vi "Loopback FPGA.vi"() -> ()   [LabVIEW 2013]
uses:
  <vilib>/Platform/TimedLoop/XDataNode/timing_clust.ctl
  <vilib>/Platform/TimedLoop/XDataNode/nitl_modes.ctl
  <vilib>/Platform/TimedLoop/XDataNode/wakeup.ctl
  <vilib>/NI/I2S-TDM IP/Controls/transmitter configuration.ctl
  <vilib>/NI/I2S-TDM IP/Controls/sync modes.ctl
  <vilib>/NI/I2S-TDM IP/Controls/receiver configuration.ctl
  <vilib>/rvi/DataTransferAndStorage/Container/Common/niFpgaContainerGetUniqueNameForEmu.vi
  <vilib>/rvi/DataTransferAndStorage/Container/Common/niFpgaContainerSetEmuInfo.vi
  <vilib>/rvi/eio/common/nirviEmuReportErrorAndStop.vi
  <vilib>/rvi/Emulation/niFpgaSctlEmulationGetInTimedLoop.vi
  <vilib>/rvi/Emulation/niFpgaEmulationReportErrorSimple.vi
  <vilib>/rvi/Emulation/niFpgaGetClockAttributes.vi
  <vilib>/rvi/Emulation/niFpgaCriticalErrorInLSC.vi
  <vilib>/rvi/DataTransferAndStorage/Container/Common/niFpgaContainerExecOnDevCompGetState.vi
  <vilib>/rvi/FIFO/Fifo_Resource/nirvififoEmulationReadFpgaImpl.vi
  <vilib>/rvi/interface/RandomDataEmulation/nirviRandomDataFPGAFIFO.vi
  <vilib>/rvi/interface/RandomDataEmulation/niFpgaRandomDataHandleErrors.vi
  <vilib>/rvi/FIFO/Fifo_Resource/nirvififoEmulationGetNumberOfElementsToReadFpgaImpl.vi
  <vilib>/rvi/FIFO/Fifo_Resource/nirvififoEmulationWriteFpgaImpl.vi
  <vilib>/rvi/FIFO/Fifo_Resource/nirvififoEmulationGetNumberOfElementsToWriteFpgaImpl.vi
  <vilib>/Platform/TimedLoop/XDataNode/XDataNode.xnode
  <vilib>/rvi/LocalResourceManager/LocalResourceManager.xnode
  <vilib>/rvi/DataTransferAndStorage/Container/XNode/niFpgaContainer.xnode
  <vilib>/rvi/FIFO/Fifo_Resource/niFpgaFifoEmulationRefIn.vi
  <vilib>/NI/I2S-TDM IP/I2S-TDM.lvlib
  <vilib>/Platform/TimedLoop/XDataNode/XDNodeRunTimeDep.lvlib
panel:
  in  "samples in":u32[](array[numeric])=[0, 0, 0, 0, 0, 0, 0, 0]
  out "receive buffer":u32
  out "signals out":cluster{"clock":bool, "sync":bool, "sdata":bool}
  out "samples out":u32[](array[numeric])
  out "transmit buffer":u32
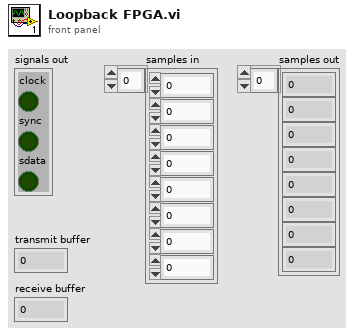
[diagram p1: front panel]
types:
  T1 = typedef "XDNodeRunTimeDep.lvlib/timing_clust.ctl" = cluster{"Expected End [f-1]":u64, "Actual End [f-1]":u64, "Finished Late? [f-1]":bool, "Expected End [i-1]":u64, "Actual End [i-1]":u64, "Finished Late? [i-1]":bool, "Expected Start [i]":u64, "Actual Start [i]":u64, "Expected Start [f]":u64, "Actual Start [f]":u64, "Source Name":string, "Structure Name":string, "Period":i64, "Deadline":i64, "Offset":i64, "Start":i64, "Priority":i32, "Timeout":i32, "Mode":T2, "Wakeup Reason":T3, "Error":errorcluster, "Source Type":string, "Secondary Source Type":string, "Global End Time":u64, "Global Start Time":u64, "Frame Duration":u64, "Iteration Duration":u64, "Assigned CPU":i32, "I/O Scan Engine Mode":u32}
  T2 = typedef "XDNodeRunTimeDep.lvlib/nitl_modes.ctl" = enum32{"No Change", "Process missed periods, maintain original phase", "Discard missed periods, maintain original phase", "Process missed periods, ignore original phase", "Discard missed periods, ignore original phase"}
  T3 = typedef "XDNodeRunTimeDep.lvlib/wakeup.ctl" = enum32{"Normal", "Aborted", "Asynchronous wakeup", "Timing source error", "Timed loop error", "Timeout"}
  T4 = typedef "I2S-TDM.lvlib/transmitter configuration.ctl" = cluster{"number of channels":u8, "bits per channel":u8, "data set edge":enum16{"rising", "falling"}, "sync mode":T5, "invert sync":bool}
  T5 = typedef "I2S-TDM.lvlib/sync modes.ctl" = enum16{"TDM - Sample Clock", "TDM - Pre-Start Pulse"}
  T6 = typedef "I2S-TDM.lvlib/receiver configuration.ctl" = cluster{"number of channels":u8, "bits per channel":u8, "data sample edge":enum16{"rising", "falling"}, "frame start delay":u8, "inverted sync":bool}
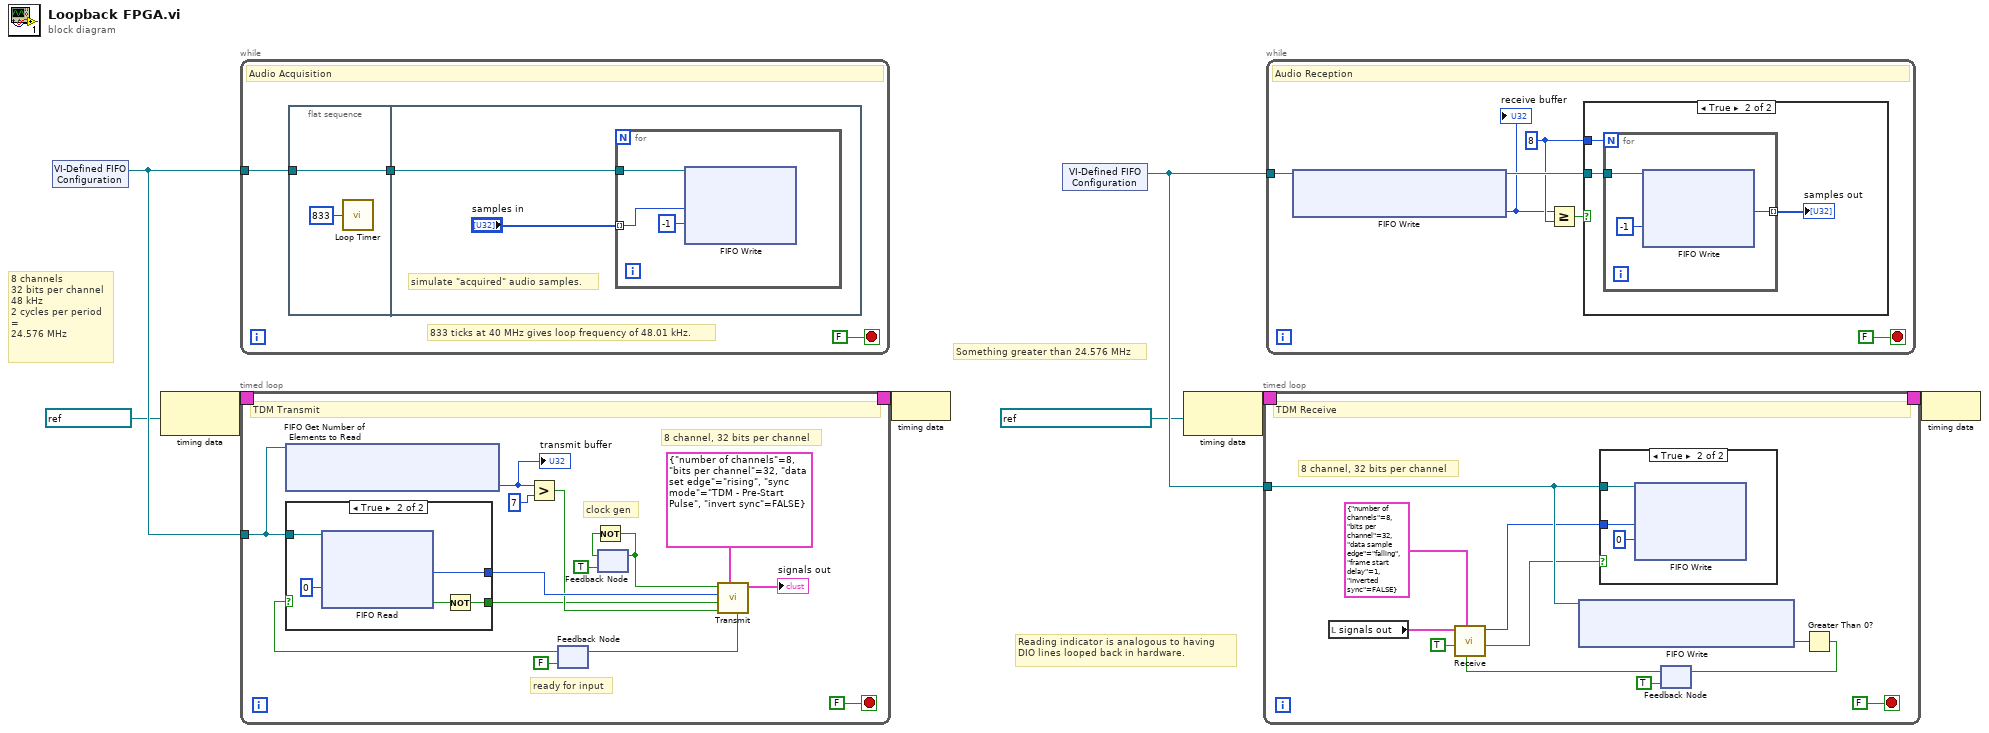
[diagram p0: block diagram]
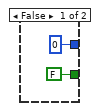
[diagram p4: hidden frame]
diagram:
  # "Reading indicator is analogous to having DIO lines looped back in hardware."
  # "Something greater than 24.576 MHz"
  # "8 channels\n32 bits per channel\n48 kHz\n2 cycles per period\n=\n24.576 MHz"
  n1 = xnode "VI-Defined FIFO Configuration"() -> ("FIFO Out"=w4:refnum<k21>)
  n2 = node-c288(refnum<k21> "24.576MHz" ("Source Name")) -> (w8:T1)
  n3 = while {
    tunnel: w4 -> [w11]
    stop <- FALSE stop-if-true
    # "833 ticks at 40 MHz gives loop frequency of 48.01 kHz."
    # "Audio Acquisition"
    n4 = flat-sequence {
      tunnel: w11 -> [w13]
      tunnel: [w13] -> w10
      tunnel: w10 -> [w15]
      frame #0 {
        n5 = call "Loop Timer"("Count(Ticks)"=u16 833) -> ()  [unwired: 1 out]
      }
      frame #1 {
        # "simulate \"acquired\" audio samples."
        n6 = for {
          tunnel: w15 -> [w18]
          tunnel: "samples in" -> [w17] mode=indexing
          n7 = xnode ("FIFO Write")("Element"=w17, "Timeout"=-1, "FIFO In"=w18) -> ()  [unwired: 2 out]
        }
      }
    }
  }
  n8 = timed-loop {
    timing: w8 -> [_]
    timing-out: [_] -> w7
    tunnel: w4 -> [w33]
    stop <- FALSE stop-if-true
    # "clock gen"
    # "8 channel, 32 bits per channel"
    # "ready for input"
    # "TDM Transmit"
    n9 = xnode ("FIFO Get Number of Elements to Read")("FIFO In"=w33) -> ("Number of Elements to Read"=w32:u32)  [unwired: 1 out]
    "transmit buffer" <- w32
    n10 = Greater?(x=w32, y=u32 7) -> (0:w24:bool)
    n11 = feedback #1(FALSE ("ready for input")) -> (w25:bool)
    n12 = case shown="True" w25 {
      tunnel: w33 -> [_ w40]
      tunnel: [u32 0 ("Element") w39] -> w28
      tunnel: [FALSE w36] -> w22
      frame False {
      }
      frame True {
        n13 = xnode ("FIFO Read")("Timeout"=0, "FIFO In"=w40) -> ("Element"=w39:u32, "Timed Out?"=w37:bool)  [unwired: 1 out]
        n14 = Not(x=w37) -> (.not. x?=w36:bool)
      }
    }
    n15 = feedback #2(TRUE) -> (w30:bool)
    n16 = Not(x=w30) -> (.not. x?=w20:bool)
    n17 = feedback-in #2(w20) -> ()
    n18 = call <vilib>:"Transmit.vi"("configuration"=T4 {"number of channels"=8, "bits per channel"=32, "data set edge"=enum."rising", "sync mode"=enum."TDM - Pre-Start Pulse", "invert sync"=FALSE}, "transmit"=w24, "input valid"=w22, "sample"=w28, "clock in"=w20) -> ("signals out"=→"signals out":cluster{"clock":bool, "sync":bool, "sdata":bool}, "ready for input"=w27:bool)  [unwired: 5 in]
    n19 = feedback-in #1(w27) -> ()
  }
  n20 = node-c288(w7) -> ()
  n21 = xnode "VI-Defined FIFO Configuration"() -> ("FIFO Out"=w2:refnum<k21>)
  n22 = node-c288(refnum<k21> "40 MHz Onboard Clock" ("Source Name")) -> (w6:T1)
  n23 = timed-loop {
    timing: w6 -> [_]
    timing-out: [_] -> w5
    tunnel: w2 -> [w49]
    stop <- FALSE stop-if-true
    # "8 channel, 32 bits per channel"
    # "TDM Receive"
    n24 = local read "signals out"() -> (w52:cluster{"clock":bool, "sync":bool, "sdata":bool})
    n25 = xnode ("FIFO Write")("FIFO In"=w49) -> ("Number of Elements to Write"=w46:u32)  [unwired: 1 out]
    n26 = feedback #3(TRUE) -> (w44:bool)
    n27 = call <vilib>:"Receive.vi"("ready for output"=w44, "configuration"=T6 {"number of channels"=8, "bits per channel"=32, "data sample edge"=enum."falling", "frame start delay"=1, "inverted sync"=FALSE}, "receive"=TRUE, "signals in"=w52) -> ("output valid"=w48:bool, "sample"=w47:u32)  [unwired: 6 in]
    n28 = case shown="True" w48 {
      tunnel: w49 -> [_ w56]
      tunnel: w47 -> [_ w54]
      frame False {
      }
      frame True {
        n29 = xnode ("FIFO Write")("Element"=w54, "Timeout"=0, "FIFO In"=w56) -> ()  [unwired: 2 out]
      }
    }
    n30 = Greater Than 0?(x=w46) -> (x > 0?=w45:bool)
    n31 = feedback-in #3(w45) -> ()
  }
  n32 = while {
    tunnel: w2 -> [w63]
    stop <- FALSE stop-if-true
    w60 = 8
    # "Audio Reception"
    n33 = xnode ("FIFO Write")("FIFO In"=w63) -> ("Number of Elements to Read"=w59:u32, "FIFO Out"=w62:refnum<k21>)
    "receive buffer" <- w59
    n34 = Greater Or Equal?(x=w59, y=w60) -> (x >= y?=w61:bool)
    n35 = case shown="True" w61 {
      tunnel: w62 -> [_ w66]
      tunnel: w60 -> [_ w65]
      frame False {
      }
      frame True {
        n36 = for {
          N: w65 -> [_]
          tunnel: w66 -> [w70]
          tunnel: [w68] -> w67 mode=indexing
          n37 = xnode ("FIFO Write")("Timeout"=-1, "FIFO In"=w70) -> ("Element"=w68:u32)  [unwired: 2 out]
        }
        "samples out" <- w67
      }
    }
  }
  n38 = node-c288(w5) -> ()
